vi "Fading_In_VI.vi"(0 "Input Array":dbl[](array[numeric]), 9 "Fading Index":i32, 11 "error in (no error)":errorcluster) -> (6 "Rising Array":dbl[](array[numeric]), 15 "error out":errorcluster)   [LabVIEW 2014]
doc: "VI zum Ausfaden eines Signals ab dem Fading Index über eine benutzerdefinierbare Länge (Fading length) [Standardwert: 400 samples]"
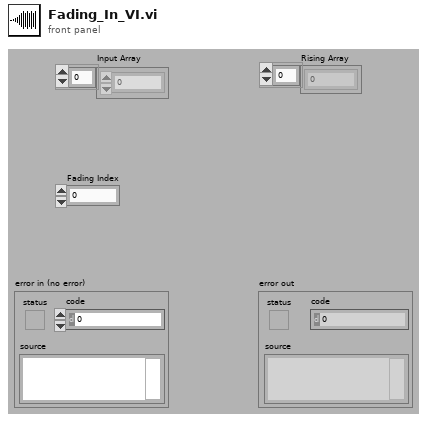
[diagram p1: front panel]
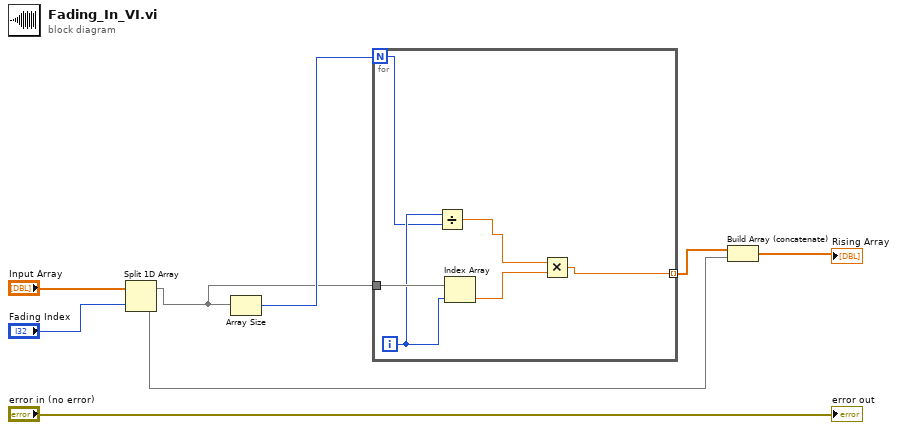
[diagram p0: block diagram]
diagram:
  n1 = Split 1D Array(array="Input Array", index="Fading Index") -> (first subarray=w3:dbl[], second subarray=w2:dbl[])
  n2 = Array Size(array=w3) -> (size(s)=w8:i32)
  n3 = for {
    N: w8 -> [w12]
    tunnel: w3 -> [w14]
    tunnel: [w9] -> w1 mode=indexing
    i -> [w13]
    n4 = Divide(x=w13, y=w12) -> (x/y=w10:dbl)
    n5 = Index Array(array=w14, index=w13) -> (element=w11:dbl)
    n6 = Multiply(x=w10, y=w11) -> (x*y=w9:dbl)
  }
  n7 = Build Array (concatenate)(w1, w2) -> (→"Rising Array":dbl[])
  "error out" <- "error in (no error)"
